vi "DP-Init DataAcq (F1L1).vi"(0 "StimGen":T3, 1 "Expt State":T5, 5 "DP stimulus params":T7={"Start (dB)"=20.0, "Stop (dB)"=80.0, "Step (dB)"=10.0, "Ear"=enum."Left", "f2 (kHz)"="", "f1"=0.0, "f1 mode"=enum."re f2", "L1"=0.0, "L1 mode"=enum."re L2"}, 7 "Init data file (T)":bool=TRUE, 9 "Avg specs":T6={"# time avgs "=8, "# spectra avgs"=4}, 11 "error in (no error)":errorcluster, 12 "Mic gain (dB)":dbl, 13 "Save waves?":bool) -> (3 "Expt State out":T5, 4 "DataAcq":T4, 15 "error out":errorcluster)   [LabVIEW 2020]
uses:
  Typedefs/DP-Stim Params (F1L1).ctl
  epl-vi-lib/Utility VIs/Type Defs/Left-Right ring.ctl
  CFTS Main Panel SubVIs/CFTS-Experiment State.ctl
  Typedefs/DP-DataAcq.ctl
  Typedefs/DP-StimGen.ctl
  Typedefs/DP Stimulus Params.ctl
  epl-vi-lib/Connection VIs/Type Defs/Input sources.ctl
panel:
  in  "DP stimulus params (old)":T1={"Start (dB)"=0.0, "Stop (dB)"=0.0, "Step (dB)"=0.0, "Ear"=enum."Left", "Mode"=enum."L1 = L2", "f2 freqs (kHz)"=""}
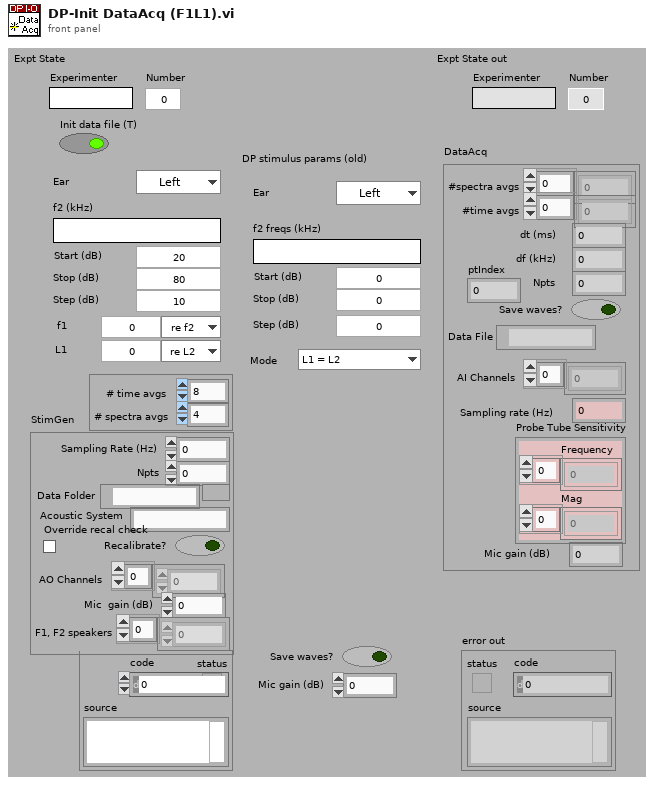
[diagram p1: front panel]
types:
  T1 = typedef "DP Stimulus Params.ctl" = cluster{"Start (dB)":dbl, "Stop (dB)":dbl, "Step (dB)":dbl, "Ear":T2, "Mode":enum16{"L1 = L2", "L1 = L2 + 10 dB"}, "f2 freqs (kHz)":string}
  T2 = typedef "Left-Right ring.ctl" = enum16{"Right", "Left"}
  T3 = typedef "DP-StimGen.ctl" = cluster{"Sampling Rate (Hz)":dbl, "Npts":i32, "Data Folder":path, "Acoustic System":string, "Recalibrate?":bool, "AO Channels":i32[], "Mic  gain (dB)":dbl, "F1, F2 speakers":i32[], "Override recal check":bool}
  T4 = typedef "DP-DataAcq.ctl" = cluster{"#spectra avgs":i32[], "#time avgs":i32[], "dt (ms)":dbl, "df (kHz)":dbl, "Npts":i32, "Save waves?":bool, "Data File":path, "AI Channels":u16[], "Sampling rate (Hz)":dbl, "Probe Tube Sensitivity":cluster{"Frequency":dbl[], "Mag":dbl[]}, "Mic gain (dB)":dbl, "ptIndex":i32}
  T5 = typedef "CFTS-Experiment State.ctl" = cluster{"Experimenter":string, "Number":u32, "Right":string, "Left":string, "Data Folder":path, "State File":path, "Version Info":string, "End Exposure Time":dbl, "Exposure Duration":string, "Run #":cluster{"CAP":i16, "ABR":i16, "DP":i16, "VsEP":i16, "MeasSeq":i16, "SubSeq":i16, "SFOAE":i16}}
  T6 = cluster{"# time avgs ":i32, "# spectra avgs":i32}
  T7 = typedef "DP-Stim Params (F1L1).ctl" = cluster{"Start (dB)":dbl, "Stop (dB)":dbl, "Step (dB)":dbl, "Ear":T2, "f2 (kHz)":string, "f1":dbl, "f1 mode":enum16{"re f2", "kHz"}, "L1":dbl, "L1 mode":enum16{"re L2", "dB"}}
  T8 = typedef "Input sources.ctl" = u16
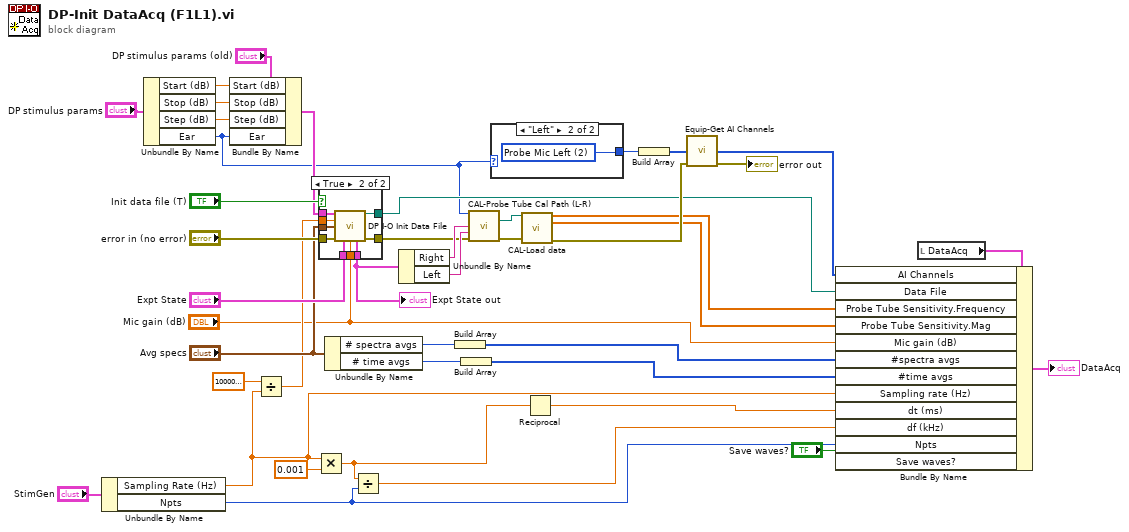
[diagram p0: block diagram]
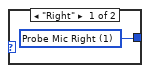
[diagram p3: hidden frame]
diagram:
  n1 = Unbundle By Name("StimGen") -> ("Sampling Rate (Hz)"=w12:dbl, "Npts"=w11:i32)
  n2 = Unbundle By Name("DP stimulus params") -> ("Start (dB)"=w6:dbl, "Stop (dB)"=w5:dbl, "Step (dB)"=w4:dbl, "Ear"=w3:T2)
  n3 = Bundle By Name(cluster="DP stimulus params (old)", "Start (dB)"=w6, "Stop (dB)"=w5, "Step (dB)"=w4, "Ear"=w3) -> (w7:T1)
  n4 = Divide(x=1000000.0, y=w12) -> (x/y=w16:dbl)
  n5 = Multiply(x=w12, y=0.001 ("x")) -> (x*y=w15:dbl)
  n6 = case shown="True" "Init data file (T)" {
    tunnel: "error in (no error)" -> [w44 w53]
    tunnel: w7 -> [_ w52]
    tunnel: "Expt State" -> [w43 w51]
    tunnel: [w44 w50] -> w35
    tunnel: [w43 w49] -> w30
    tunnel: [_ w48] -> w24
    tunnel: "Avg specs" -> [_ w47]
    tunnel: w16 -> [_ w46]
    tunnel: "Mic gain (dB)" -> [_ w45]
    frame False {
    }
    frame True {
      n7 = call "DP I-O Init Data File.vi"("DP stimulus params"=w52, "Sampling interval (us)"=w46, "Averaging Specs"=w47, "error in (no error)"=w53, "Expt State"=w51, "Probe Mic Gain (dB)"=w45) -> ("Path"=w48:path, "Expt State out"=w49:T5, "error out"=w50:errorcluster)  [unwired: 7 in]
    }
  }
  "Expt State out" <- w30
  n8 = Unbundle By Name("Avg specs") -> ("# spectra avgs"=w21:i32, "# time avgs"=w20:i32)
  n9 = Divide(x=w15, y=w11) -> (x/y=w18:dbl)
  n10 = Unbundle By Name(w30) -> ("Right"=w37:string, "Left"=w36:string)
  n11 = Build Array(w21) -> (w2:i32[])
  n12 = Build Array(w20) -> (w1:i32[])
  n13 = call "CAL-Probe Tube Cal Path (L-R).vi"("Ear"=w3, "Right"=w37, "Left"=w36, "error in (no error)"=w35) -> ("Probe Tube Cal Path"=w33:path, "error out"=w34:errorcluster)  [unwired: 10 in]
  n14 = case shown="\"Left\"" w3 {
    tunnel: [w54 w55] -> w42
    frame "Right" {
      w54 = T8 1 items=["--unused--", "Probe Mic Right", "Probe Mic Left", "Cal Mic", "ABR", "CAP Right", "CAP Left", "Startle piezo", "Temperature", "Heart rate"] ("Ring")
    }
    frame "Left" {
      w55 = T8 2 items=["--unused--", "Probe Mic Right", "Probe Mic Left", "Cal Mic", "ABR", "CAP Right", "CAP Left", "Startle piezo", "Temperature", "Heart rate"] ("Ring")
    }
  }
  n15 = call "CAL-Load data.vi"("user path"=w33, "error in (no error)"=w34) -> ("Frequency (Hz)"=w27:dbl[], "Mag"=w26:dbl[], "error out"=w29:errorcluster)  [unwired: 6 in, 5 out]
  n16 = Reciprocal(x=w15) -> (1/x=w14:dbl)
  n17 = Build Array(w42) -> (w41:T8[])
  n18 = call "Equip-Get AI Channels.vi"("Inputs"=w41, "error in (no error)"=w29) -> ("AI Channels"=w25:i32[], "error out"=→"error out":errorcluster)  [unwired: 12 in]
  n19 = local read "DataAcq"() -> (w32:T4)
  n20 = Bundle By Name(cluster=w32, "AI Channels"=w25, "Data File"=w24, "Probe Tube Sensitivity.Frequency"=w27, "Probe Tube Sensitivity.Mag"=w26, "Mic gain (dB)"="Mic gain (dB)", "#spectra avgs"=w2, "#time avgs"=w1, "Sampling rate (Hz)"=w12, "dt (ms)"=w14, "df (kHz)"=w18, "Npts"=w11, "Save waves?"="Save waves?") -> (→"DataAcq":T4)
